vi "0xE0 Запрос количества доступных параметров (SubVI).vi"(11 "String in":string) -> (3 "String out":string)   [LabVIEW 2017, in "LV_Unicorn.lvlib"]
uses:
  LV_Unicorn.lvlib
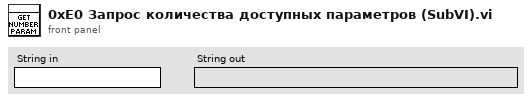
[diagram p1: front panel]
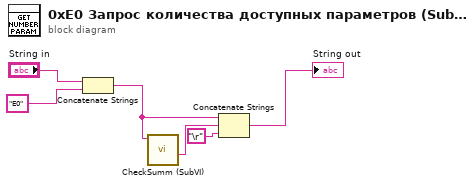
[diagram p0: block diagram]
diagram:
  n1 = Concatenate Strings("String in", "E0" ("string")) -> (w1:string)
  n2 = call "CheckSumm (SubVI).vi"("Input String"=w1) -> ("CheckSumm"=w2:string)  [unwired: 7 in, 3 out]
  n3 = Concatenate Strings(w1, w2, "\r") -> (→"String out":string)
